vi "fgv_MovCor setup.vi"(8 "error in (no error)":errorcluster, 10 "Status":enum16{"Initialize", "Write", "Read"}(ring), 11 "MovCor Cluster":T1={"x_offset_host"=0.0, "y_offset_host"=0.0, "use host offset"=TRUE, "Set_Ref_Centroid"=FALSE, "OldChirpCode"=FALSE, "use array of offsets"=FALSE, "x_offset_host array"=[], "y_offset_host array "=[], "use host offset Z"=TRUE, "swap Z"=FALSE, "z_offset_host "=0.0}) -> (0 "error out":errorcluster, 3 "MovCor Cluster":T1={"x_offset_host"=0.0, "y_offset_host"=0.0, "use host offset"=TRUE, "Set_Ref_Centroid"=FALSE, "OldChirpCode"=FALSE, "use array of offsets"=TRUE, "x_offset_host array"=[], "y_offset_host array "=[], "use host offset Z"=TRUE, "swap Z"=FALSE, "z_offset_host "=0.0})   [LabVIEW 2020]
uses:
  Typedefs/test_fpga_control.ctl
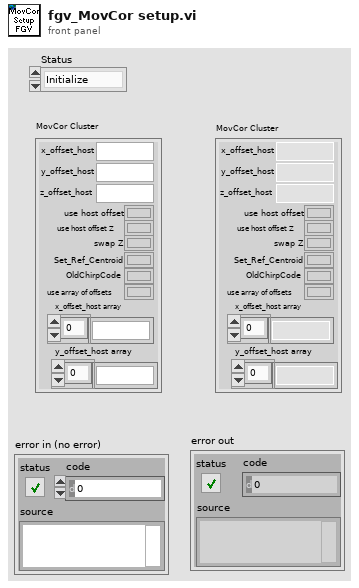
[diagram p1: front panel]
types:
  T1 = typedef "test_fpga_control.ctl" = cluster{"x_offset_host":fxp<+/-,16,8>, "y_offset_host":fxp<+/-,16,8>, "use host offset":bool, "Set_Ref_Centroid":bool, "OldChirpCode":bool, "use array of offsets":bool, "x_offset_host array":fxp<+/-,16,8>[], "y_offset_host array ":fxp<+/-,16,8>[], "use host offset Z":bool, "swap Z":bool, "z_offset_host ":fxp<+/-,16,8>}
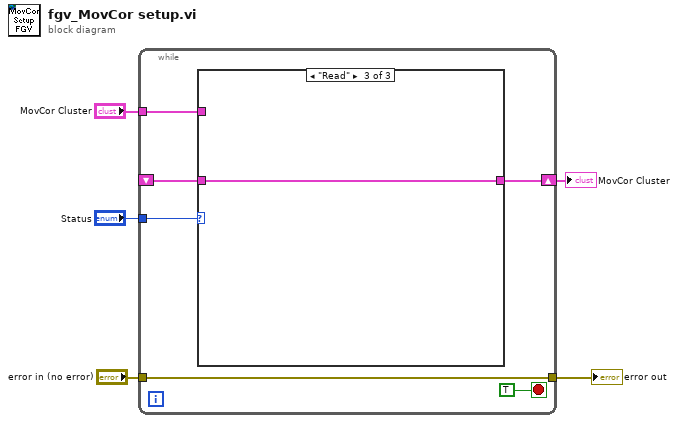
[diagram p0: block diagram]
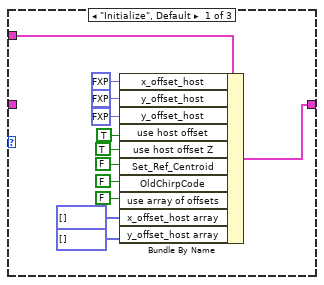
[diagram p2: hidden frame]
diagram:
  n1 = while {
    tunnel: "Status" -> [w10]
    shift-right: [w9] -> w3
    shift-left: _ -> [w8]
    tunnel: "MovCor Cluster" -> [w7]
    tunnel: "error in (no error)" -> [w6]
    tunnel: [w6] -> w1
    stop <- TRUE stop-if-true
    n2 = case shown="\"Read\"" w10 {
      tunnel: [w23 w24 w25] -> w9
      tunnel: w8 -> [_ _ w25]
      tunnel: w7 -> [w22 w24 _]
      frame "Initialize", Default {
        n3 = Bundle By Name(cluster=w22, "x_offset_host"=fxp<+/-,16,8> 0.0, "y_offset_host"=fxp<+/-,16,8> 0.0, "y_offset_host"=fxp<+/-,16,8> 0.0, "use host offset"=TRUE, "use host offset Z"=TRUE, "Set_Ref_Centroid"=FALSE, "OldChirpCode"=FALSE, "use array of offsets"=FALSE, "x_offset_host array"=fxp<+/-,16,8>[] [], "y_offset_host array"=fxp<+/-,16,8>[] []) -> (w23:T1)
      }
      frame "Write" {
      }
      frame "Read" {
      }
    }
  }
  "MovCor Cluster" <- w3
  "error out" <- w1
